vi "WILT Create Start Button Array.vi"(11 "Start Buttons Cluster":T1) -> (2 "Station Number":i32, 3 "Start Button Array":bool[](array[boolean]), 5 "Valve Found!!":bool)   [LabVIEW 2016]
uses:
  Type Definitions/WILT Start Button Cluster.ctl
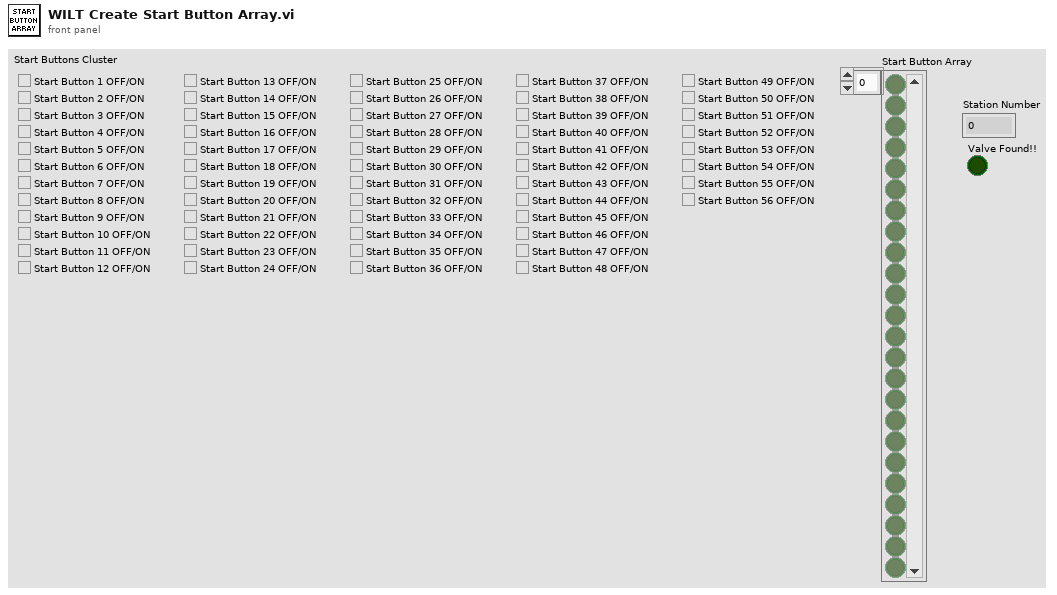
[diagram p1: front panel]
types:
  T1 = typedef "WILT Start Button Cluster.ctl" = cluster{"Start Button 21":bool, "Start Button 22":bool, "Start Button 23":bool, "Start Button 24":bool, "Start Button 25":bool, "Start Button 26":bool, "Start Button 27":bool, "Start Button 28":bool, "Start Button 29":bool, "Start Button 30":bool, "Start Button 31":bool, "Start Button 32":bool, "Start Button 33":bool, "Start Button 34":bool, "Start Button 35":bool, "Start Button 36":bool, "Start Button 37":bool, "Start Button 38":bool, "Start Button 39":bool, "Start Button 40":bool, "Start Button 41":bool, "Start Button 42":bool, "Start Button 43":bool, "Start Button 44":bool, "Start Button 12":bool, "Start Button 11":bool, "Start Button 10":bool, "Start Button 9":bool, "Start Button 8":bool, "Start Button 7":bool, "Start Button 6":bool, "Start Button 5":bool, "Start Button 4":bool, "Start Button 3":bool, "Start Button 2":bool, "Start Button 1":bool, "Start Button 20":bool, "Start Button 19":bool, "Start Button 18":bool, "Start Button 17":bool, "Start Button 16":bool, "Start Button 15":bool, "Start Button 14":bool, "Start Button 13":bool, "Start Button 45":bool, "Start Button 46":bool, "Start Button 47":bool, "Start Button 48":bool, "Start Button 49":bool, "Start Button 50":bool, "Start Button 51":bool, "Start Button 52":bool, "Start Button 53":bool, "Start Button 54":bool, "Start Button 55":bool, "Start Button 56":bool}
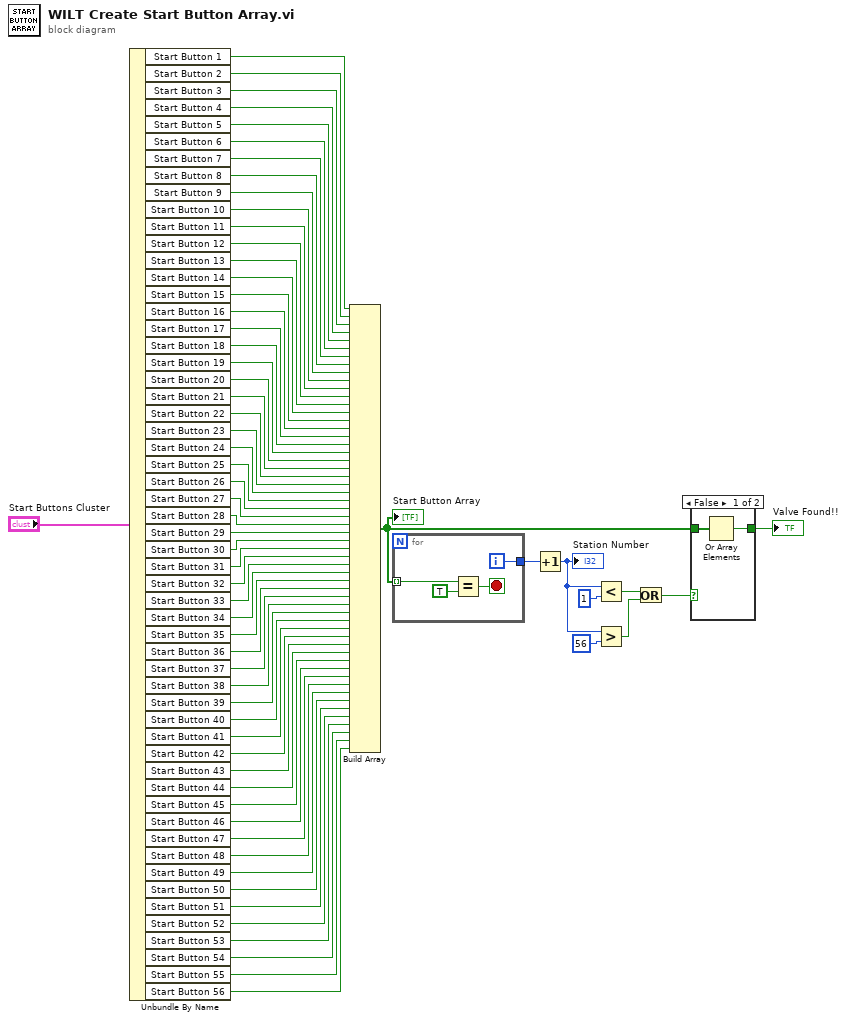
[diagram p0: block diagram]
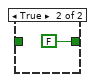
[diagram p2: hidden frame]
diagram:
  n1 = Unbundle By Name("Start Buttons Cluster") -> ("Start Button 1"=w22:bool, "Start Button 2"=w23:bool, "Start Button 3"=w24:bool, "Start Button 4"=w25:bool, "Start Button 5"=w26:bool, "Start Button 6"=w27:bool, "Start Button 7"=w28:bool, "Start Button 8"=w29:bool, "Start Button 9"=w30:bool, "Start Button 10"=w31:bool, "Start Button 11"=w32:bool, "Start Button 12"=w33:bool, "Start Button 13"=w34:bool, "Start Button 14"=w35:bool, "Start Button 15"=w36:bool, "Start Button 16"=w37:bool, "Start Button 17"=w38:bool, "Start Button 18"=w39:bool, "Start Button 19"=w40:bool, "Start Button 20"=w41:bool, "Start Button 21"=w65:bool, "Start Button 22"=w64:bool, "Start Button 23"=w63:bool, "Start Button 24"=w62:bool, "Start Button 25"=w61:bool, "Start Button 26"=w60:bool, "Start Button 27"=w59:bool, "Start Button 28"=w58:bool, "Start Button 29"=w57:bool, "Start Button 30"=w56:bool, "Start Button 31"=w55:bool, "Start Button 32"=w54:bool, "Start Button 33"=w53:bool, "Start Button 34"=w52:bool, "Start Button 35"=w51:bool, "Start Button 36"=w50:bool, "Start Button 37"=w49:bool, "Start Button 38"=w48:bool, "Start Button 39"=w47:bool, "Start Button 40"=w46:bool, "Start Button 41"=w45:bool, "Start Button 42"=w44:bool, "Start Button 43"=w43:bool, "Start Button 44"=w42:bool, "Start Button 45"=w21:bool, "Start Button 46"=w20:bool, "Start Button 47"=w19:bool, "Start Button 48"=w18:bool, "Start Button 49"=w17:bool, "Start Button 50"=w16:bool, "Start Button 51"=w15:bool, "Start Button 52"=w14:bool, "Start Button 53"=w13:bool, "Start Button 54"=w12:bool, "Start Button 55"=w11:bool, "Start Button 56"=w10:bool)
  n2 = Build Array(w22, w23, w24, w25, w26, w27, w28, w29, w30, w31, w32, w33, w34, w35, w36, w37, w38, w39, w40, w41, w65, w64, w63, w62, w61, w60, w59, w58, w57, w56, w55, w54, w53, w52, w51, w50, w49, w48, w47, w46, w45, w44, w43, w42, w21, w20, w19, w18, w17, w16, w15, w14, w13, w12, w11, w10) -> (w8:bool[])
  "Start Button Array" <- w8
  n3 = for {
    tunnel: w8 -> [w70] mode=indexing
    tunnel: [w67] -> w9
    i -> [w67]
    stop <- w68 stop-if-true
    n4 = Equal?(x=w70, y=TRUE) -> (x = y?=w68:bool)
  }
  n5 = Increment(x=w9) -> (x+1=w3:i32)
  "Station Number" <- w3
  n6 = Less?(x=w3, y=1) -> (x < y?=w5:bool)
  n7 = Greater?(x=w3, y=56) -> (0:w4:bool)
  n8 = Or(x=w5, y=w4) -> (x .or. y?=w1:bool)
  n9 = case shown="False" w1 {
    tunnel: w8 -> [w72 _]
    tunnel: [w71 FALSE] -> w7
    frame False {
      n10 = Or Array Elements(Boolean array=w72) -> (logical OR=w71:bool)
    }
    frame True {
    }
  }
  "Valve Found!!" <- w7
